vi "Set panel size and  place center.vi"(0 "Path":path, 1 "Close Reference (false)":bool, 5 "Panel Width":i32, 7 "Panel Height":i32, 9 "FP.Origin in(H & V)":cluster{"Horizontal":i16, "Vertical":i16}, 11 "error in (no error)":errorcluster, 12 "Set (false)":bool) -> (4 "Application or VI Refnum":refnum<vi>, 6 "FP.Origin out(H & V)":cluster{"Horizontal":i16, "Vertical":i16}, 8 "FP.WinBounds":T2, 10 "FP.PanelBounds":T1, 15 "error out":errorcluster)   [LabVIEW 2016]
doc: "This VI is used to set the panel size and plce it in the center of the window current"
uses:
  <vilib>/Utility/miscctls.llb/LVRectTypeDef.ctl
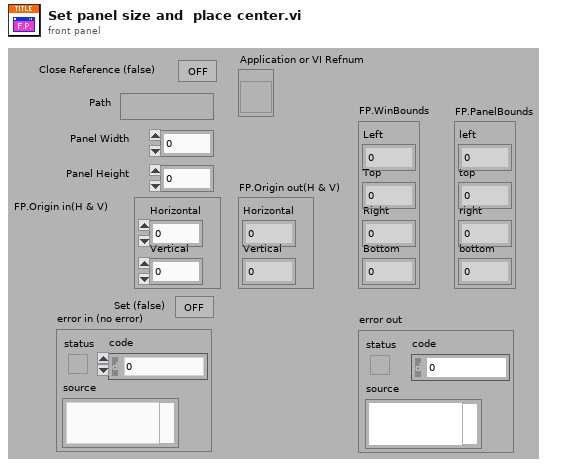
[diagram p1: front panel]
types:
  T1 = cluster{"left":i16, "top":i16, "right":i16, "bottom":i16}
  T2 = typedef "LVRectTypeDef.ctl" = cluster{"Left":i16, "Top":i16, "Right":i16, "Bottom":i16}
  T3 = typedef "LVAllMonitorsDisplayTypeDef.ctl" = cluster{"Bounds":cluster{"Left":i16, "Top":i16, "Right":i16, "Bottom":i16}, "Depth":i16}[]
  T4 = cluster{"Bounds":cluster{"Left":i16, "Top":i16, "Right":i16, "Bottom":i16}, "Depth":i16}
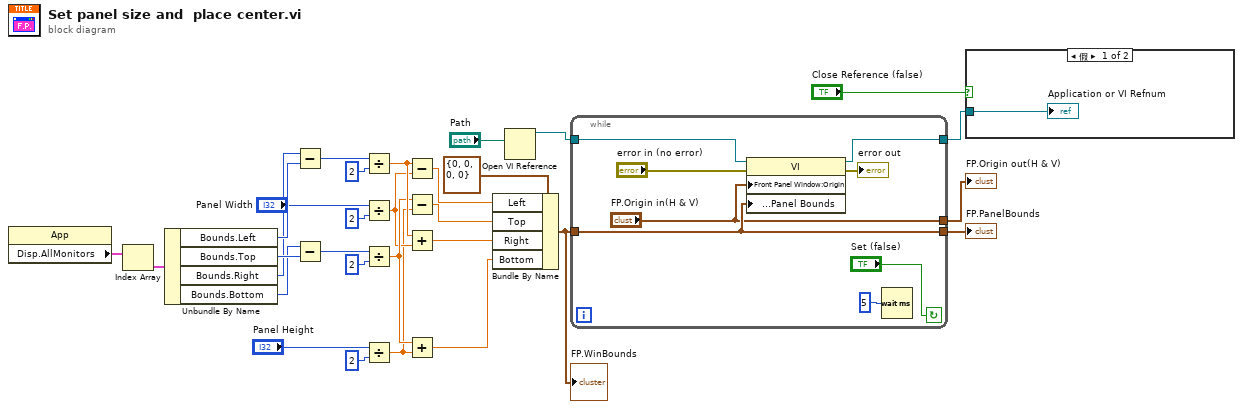
[diagram p0: block diagram]
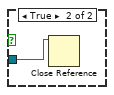
[diagram p2: hidden frame]
diagram:
  n1 = property class="App"() -> ("Disp.AllMonitors"=w2:T3)  [unwired: 2 in, 2 out]
  n2 = Index Array(array=w2) -> (element=w1:T4)  [unwired: 1 in]
  n3 = Unbundle By Name(w1) -> ("Bounds.Left"=w30:i16, "Bounds.Top"=w29:i16, "Bounds.Right"=w28:i16, "Bounds.Bottom"=w27:i16)
  n4 = Subtract(x=w28, y=w30) -> (x-y=w26:i16)
  n5 = Subtract(x=w27, y=w29) -> (x-y=w24:i16)
  n6 = Divide(x=w26, y=i16 2) -> (x/y=w18:dbl)
  n7 = Divide(x="Panel Width", y=2) -> (x/y=w16:dbl)
  n8 = Divide(x=w24, y=i16 2) -> (x/y=w17:dbl)
  n9 = Divide(x="Panel Height", y=2) -> (x/y=w15:dbl)
  n10 = Subtract(x=w18, y=w16) -> (x-y=w14:dbl)
  n11 = Subtract(x=w17, y=w15) -> (x-y=w12:dbl)
  n12 = Add(x=w18, y=w16) -> (x+y=w11:dbl)
  n13 = Add(x=w17, y=w15) -> (x+y=w13:dbl)
  n14 = Bundle By Name(cluster=T2 {"Left"=0, "Top"=0, "Right"=0, "Bottom"=0} ("显示:主工作区"), "Left"=w14, "Top"=w12, "Right"=w11, "Bottom"=w13) -> (w6:T2)
  "FP.WinBounds" <- w6
  n15 = Open VI Reference(vi path="Path") -> (vi reference=w10:refnum<vi>)  [unwired: 5 in, 1 out]
  n16 = while {
    tunnel: [w38] -> w7
    tunnel: w10 -> [w37]
    tunnel: ["FP.Origin in(H & V)"] -> w5
    tunnel: [w32] -> w4
    tunnel: w6 -> [w32]
    stop <- "Set (false)" continue-if-true
    n17 = property class="VI"(reference=w37, error in="error in (no error)", "Front Panel Window:Origin"="FP.Origin in(H & V)", "Front Panel Window:Panel Bounds"=w32) -> (reference out=w38:refnum<vi>, error out=→"error out":errorcluster)
    n18 = Wait (ms)(milliseconds to wait=u32 5) -> ()  [unwired: 1 out]
  }
  "FP.Origin out(H & V)" <- w5
  "FP.PanelBounds" <- w4
  n19 = case shown="假" "Close Reference (false)" {
    tunnel: w7 -> [w39 w40]
    frame False {
      "Application or VI Refnum" <- w39
    }
    frame True {
      n20 = Close Reference(reference=w40) -> ()  [unwired: 1 in, 1 out]
    }
  }
